vi "ASE Control Experiment Week2.vi"() -> ()   [LabVIEW 2018]
uses:
  <vilib>/Simulation/Scripting/Companion Diagram/SimConfigNode/SimParams.ctl
  <vilib>/Simulation/Scripting/Companion Diagram/SimConfigNode/_simSolvers.ctl
  <vilib>/Simulation/Implementation/Shared/SIMSCR Execution Mode.ctl
  <vilib>/Platform/TimedLoop/XDataNode/timing_clust.ctl
  <vilib>/Platform/TimedLoop/XDataNode/nitl_modes.ctl
  <vilib>/Platform/TimedLoop/XDataNode/wakeup.ctl
  <vilib>/Simulation/Param Hierarchy/Typedefs/SIMPH Param Control Actions.ctl
  <vilib>/Simulation/Implementation/Shared/SIM limit type.ctl
  <vilib>/Simulation/Scripting/Editor Utilities/SIM subVI tag data.ctl
  <vilib>/Simulation/Scripting/Editor Utilities/SIM subVI execution type.ctl
  <vilib>/Simulation/Implementation/Shared/NILVSim_ParamChanged.vi
  <vilib>/Simulation/Implementation/Shared/NILVSim_FinishedLate.vi
  <vilib>/Simulation/Implementation/Shared/NILVSIM_BeginStep.vi
  <vilib>/Simulation/Utility/Implementation/SIM Halt.vi
  <vilib>/Simulation/DataSources/Implementation/NILVSim Signal Generator.llb/SIM Signal Generator (scalar).vi
  <vilib>/Simulation/Nonlinear/Implementation/NILVSim Saturation.llb/SIM Saturation (scalar).vi
  <vilib>/Simulation/Utility/Implementation/NILVSim Memory.llb/NILVSim Memory (core).vi
  <vilib>/Simulation/ContinuousLinear/Implementation/NILVSim Transfer Function.llb/SIM Transfer Function Distributor (SISO).vi
  <vilib>/Simulation/SignalArithmetic/Implementation/NILVSim Gain.llb/SIM Gain (scalar).vi
  <vilib>/Simulation/ContinuousLinear/Implementation/NILVSim Integrator new.llb/SIM Integrator distributor (scalar).vi
  <vilib>/Simulation/ContinuousLinear/Implementation/NILVSim Transfer Function.llb/SIM Transfer Function Collector (SISO).vi
  <vilib>/Simulation/Nonlinear/Implementation/NILVSim RateLimiter.llb/SIM RateLimiter (scalar).vi
  <vilib>/Simulation/Implementation/Shared/SIM Fire Discrete SubVI.vi
  <vilib>/Simulation/ContinuousLinear/Implementation/NILVSim Transfer Function Direct.llb/SIM Transfer Function Direct (SISO).vi
  <vilib>/Simulation/ContinuousLinear/Implementation/NILVSim Derivative.llb/SIM derivative (scalar).vi
  <vilib>/Simulation/ContinuousLinear/Implementation/NILVSim Integrator new.llb/SIM Integrator collector (scalar).vi
  <vilib>/Simulation/SignalArithmetic/Implementation/NILVSim Gain.llb/SIM Gain (vector).vi
  <vilib>/Simulation/SignalArithmetic/Implementation/NILVSim Gain.llb/SIM Gain (dot product).vi
  <vilib>/Simulation/Nonlinear/Implementation/NILVSim Saturation.llb/SIM Saturation (vector).vi
  <vilib>/Simulation/Implementation/Shared/NILVSim_Manager.vi
  <vilib>/Utility/error.llb/Clear Errors.vi
  <vilib>/Simulation/Implementation/Shared/NILVSim_FinalizeModel.vi
  <vilib>/Simulation/Implementation/Shared/SIM Fire Discrete SubVI (Core).vi
  <vilib>/addons/Control Design/_Model Construction/Model Creation.llb/Model Creation SubVI/cd_Create State Space Model.vi
  <vilib>/FPGAPlugInAG/cRIO-9068/niLvFpga_Open_cRIO-9068.vi
  <vilib>/rvi/interface/common/dynamic/niFpgaDynamicAddResources.vi
  <vilib>/Simulation/Implementation/Shared/SIM Unbundle Sim Info.vi
  <vilib>/Simulation/Implementation/Shared/SIMSH Read Queue.vi
  <vilib>/Simulation/Implementation/Shared/NILVSim_Initialize.vi
  <vilib>/Utility/error.llb/Error Cluster From Error Code.vi
  <vilib>/rvi/errors/niLvFpgaAdjustHostInterfaceError.vi
  <vilib>/Simulation/Utility/Implementation/NILVSim Get Time and IsAcceptedStep.vi
  <vilib>/Simulation/Implementation/Shared/NILVSim_GetModelError.vi
  <vilib>/Simulation/Implementation/Shared/SIM Bundle Sim Info.vi
  <vilib>/FPGAPlugInAG/Dynamic/niLvFpga_Close_Dynamic.vi
  <vilib>/rvi/interface/nirviOpenFPGA/nirviOpenFPGA.xnode
  Week 1 - Direct State Feedback/FPGA Bitfiles/BasicLinearContr_FPGATarget_FPGAQ1MODULE2_5Qds2sFCJDU.lvbitx
  FPGA_Q1_MODULE.vi
  <vilib>/Simulation/Scripting/Companion Diagram/SimConfigNode/SimDog.xnode
  <vilib>/Quanser/Rapid Control Prototyping Toolkit/discrete/_TypeSpecific/CL Bias Removal (Scalar).vi
  <vilib>/Quanser/Rapid Control Prototyping Toolkit/discrete/CL Bias Removal.vi
  <vilib>/addons/Control Design/_Implementation/CD Continuous Observer.vi
  <vilib>/Platform/TimedLoop/XDataNode/XDataNode.xnode
  <vilib>/rvi/interface/nirviReadWriteControl/nirviReadWriteControl.xnode
  <vilib>/Simulation/Implementation/XNodeFramework/SimXNode/SimX.xnode
  <vilib>/rvi/interface/nirviCloseFPGA/nirviCloseFPGA.xnode
  <vilib>/rvi/interface/Simulation/niFpgaSimulationCallBeginRW.vi
  <vilib>/Simulation/ContinuousLinear/Implementation/NILVSim Transfer Function.llb/SIM Transfer Function (SISO).vi
  <vilib>/Simulation/ContinuousLinear/Implementation/NILVSim Integrator new.llb/SIM Integrator (scalar).vi
  NiFpgaLv.dll
  <vilib>/addons/Control Design/_Model Construction/NI_LinSys_Model Creation.lvlib
  <vilib>/Platform/TimedLoop/XDataNode/XDNodeRunTimeDep.lvlib
  <vilib>/Simulation/Implementation/Shared/NI_SIM_Implementation.lvlib
panel:
  in  "Observer Gain":dbl[][](array[numeric])=[[0.0]]
  out "2":T1(graph)
  out "?":cluster{"output y(t)":dbl, "output y(t)":dbl}(graph)
  out "Active Suspension Motor Voltage (V) 2":dbl(graph)
  in  "gain":dbl[](array[numeric])=[1.0]
  in  "Enable active suspension":bool
  out "Zr(m), Zs(m), Zus(m)":T2(graph)={"output"=0.0096065956, "Result"=0.0090666584, "output"=0.0091514816}
  in  "Setpoint Command":T3={"Amplitude (m)"=0.01, "Frequency (Hz)"=0.3} caption="Road (Bottom Plate)\nAmplitude Command (m)" {"Frequency (Hz)" min=0.0 max=0.5 step=0.009999999776482582 format="%_3f"; "Amplitude (m)" min=-10.0 max=10.0 step=0.5 format="%_3f"}
  out "Active Suspension Motor Voltage (V)":dbl(graph)
  out "Accelerometer Signal":dbl(graph)
  in  "Halt?":bool
  in  "Enable motor":bool
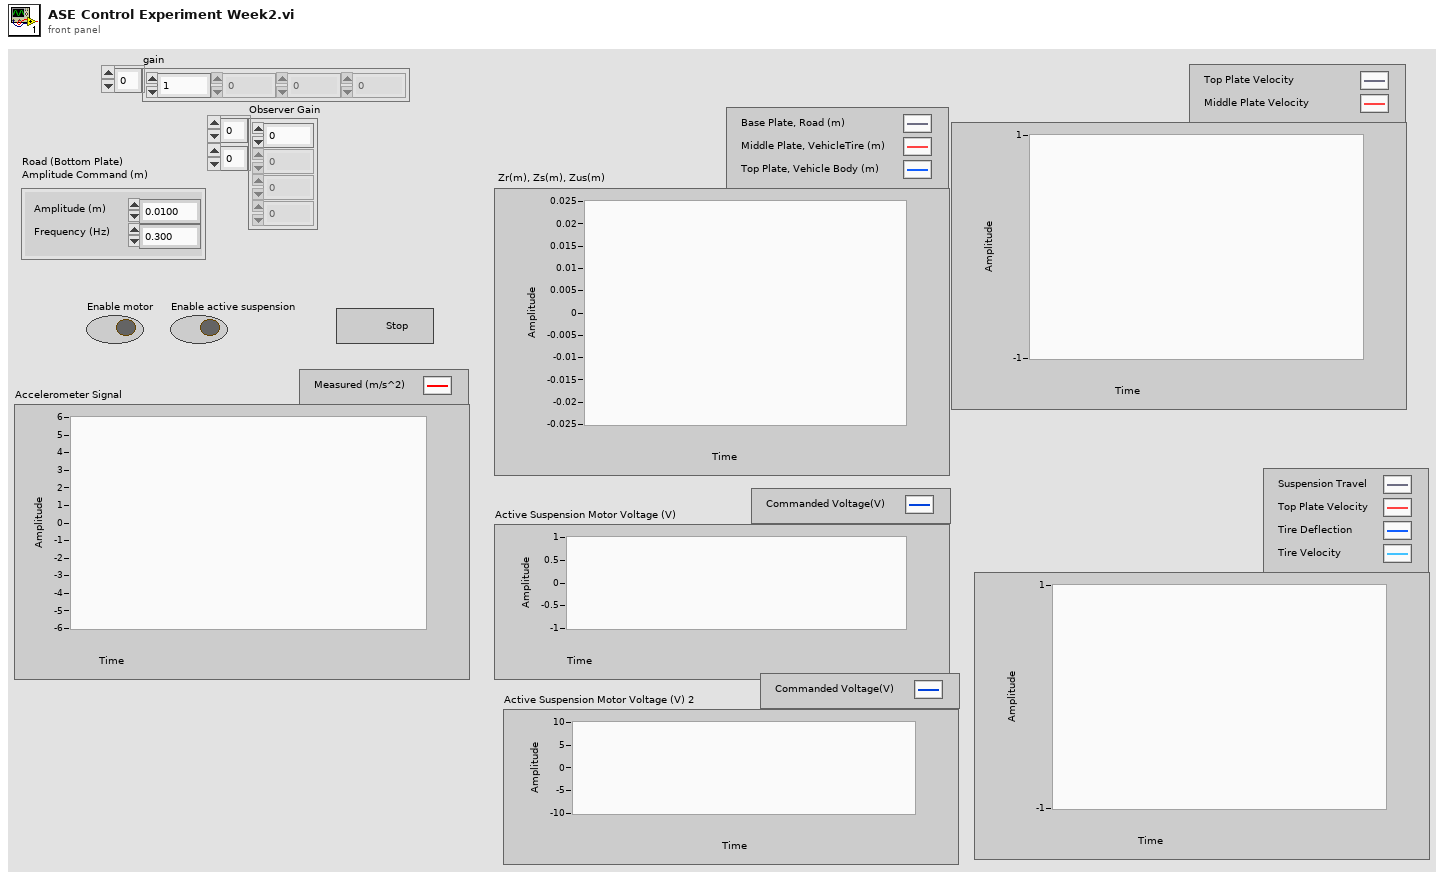
[diagram p1: front panel]
types:
  T1 = cluster{"Estimated State xhat(t)[0]":dbl, "Estimated State xhat(t)[1]":dbl, "Estimated State xhat(t)[2]":dbl, "Estimated State xhat(t)[3]":dbl, "Estimated State xhat(t)[4]":dbl, "Estimated State xhat(t)[5]":dbl, "Estimated State xhat(t)[6]":dbl, "Estimated State xhat(t)[7]":dbl, "Estimated State xhat(t)[8]":dbl}
  T2 = cluster{"output":dbl, "Result":dbl, "output":dbl}
  T3 = cluster{"Amplitude (m)":dbl, "Frequency (Hz)":dbl}
  T4 = typedef "NI_LinSys_Model Typedefs.lvlib/CD State Space Model (MIMO).ctl" = cluster{"properties":T5, "A":dbl[][], "B":dbl[][], "C":dbl[][], "D":dbl[][], "StateNames":string[], "Transport Delay":dbl[][]}
  T5 = typedef "NI_LinSys_Model Typedefs.lvlib/CD General Elements.ctl" = cluster{"Model name":string, "Input names":string[], "Output names":string[], "Input Delays":dbl[], "Output Delays":dbl[], "Sampling Time":dbl, "Notes":string}
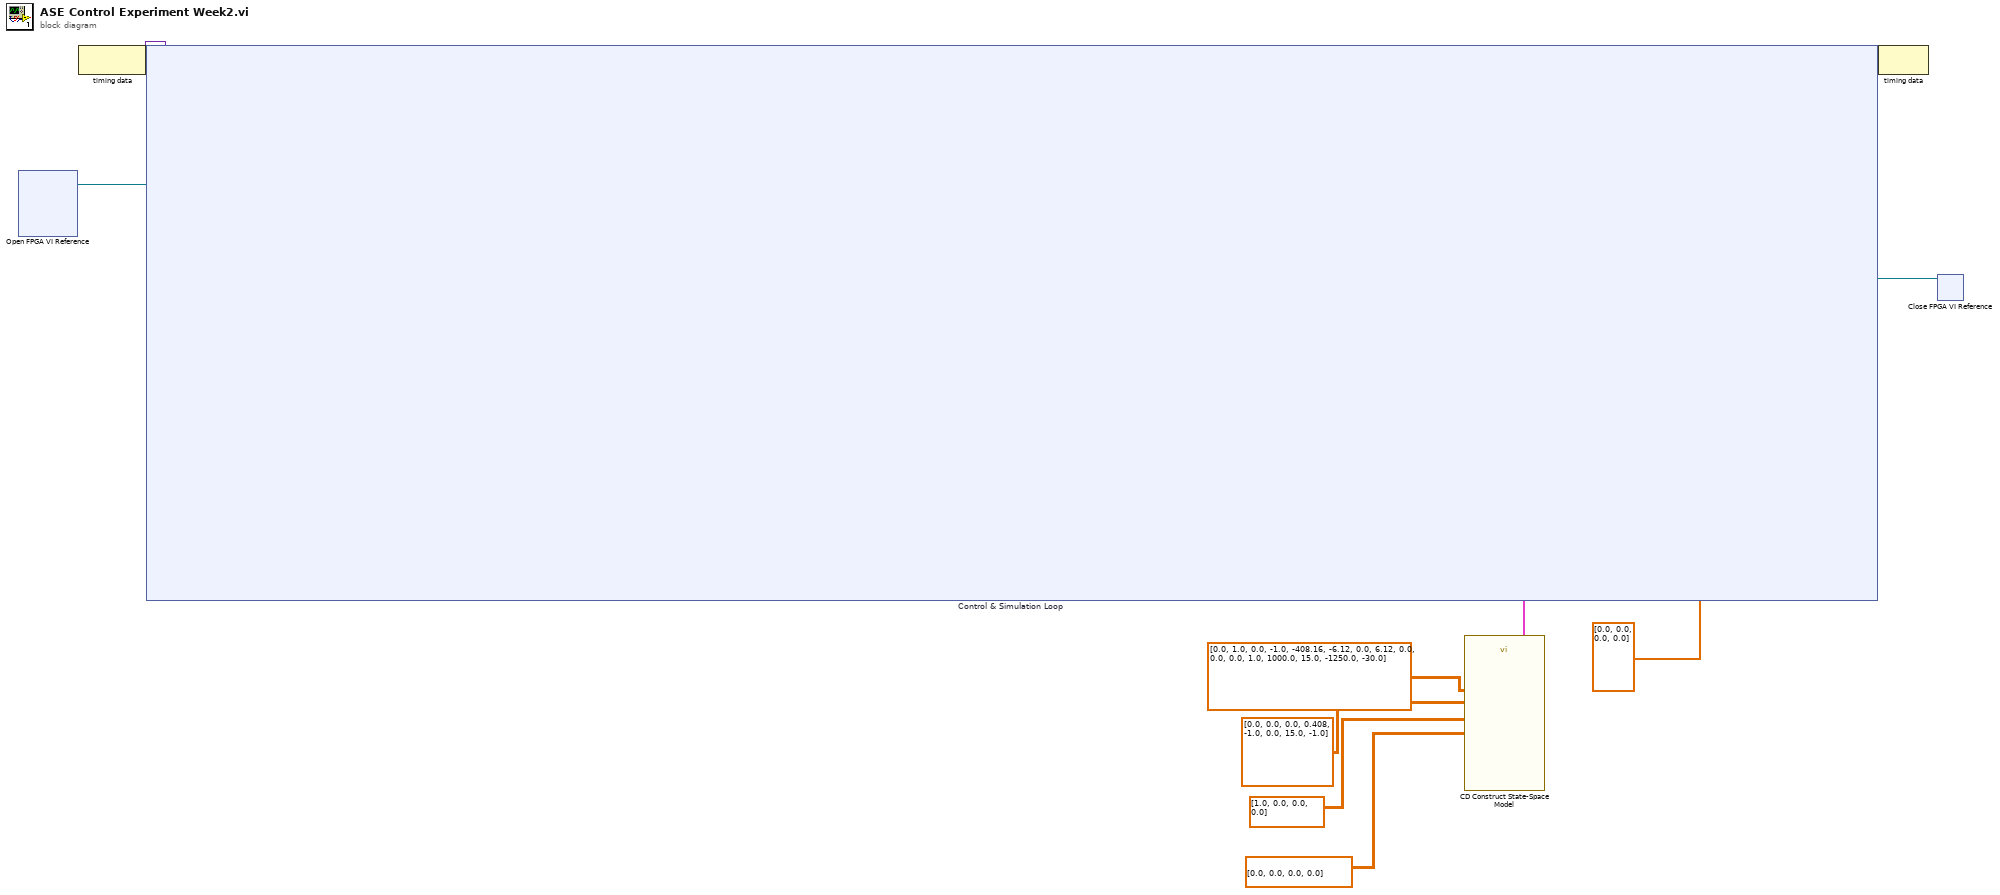
[diagram p0: block diagram]
diagram:
  n1 = xnode "Open FPGA VI Reference"() -> ("FPGA VI Reference Out"=w7:refnum<k20>)  [unwired: 2 in, 1 out]
  n2 = node-c288() -> (w10:variant)  [unwired: 1 in]
  n3 = call-poly <vilib>:"CD Construct State-Space Model.vi"("A"=dbl[][] [[0.0, 1.0, 0.0, -1.0], [-408.16, -6.12, 0.0, 6.12], [0.0, 0.0, 0.0, 1.0], [1000.0, 15.0, -1250.0, -30.0]], "B"=dbl[][] [[0.0, 0.0], [0.0, 0.408], [-1.0, 0.0], [15.0, -1.0]], "C"=dbl[][] [[1.0, 0.0, 0.0, 0.0]], "D"=dbl[][] [[0.0, 0.0], [0.0, 0.0]]) -> ("State-Space Model"=w6:T4)  [unwired: 10 in, 1 out]
  n4 = node-c254 "Control & Simulation Loop"(w10, w7, w6, dbl[] [0.0, 0.0, 0.0, 0.0]) -> (w9:variant, w8:refnum<k20>)
  n5 = node-c288(w9) -> ()  [unwired: 1 out]
  n6 = xnode "Close FPGA VI Reference"("FPGA VI Reference In"=w8) -> ()  [unwired: 1 in, 1 out]
